vi "Host_ZConstantCurrentOscillation.vi"() -> ()   [LabVIEW 2014]
uses:
  <vilib>/Native 3D Graph/xcontrol/3DPC_SurfacePlot.xctl
  <vilib>/FPGAPlugInAG/PCIe-7851R/niLvFpga_Open_PCIe-7851R.vi
  <vilib>/rvi/interface/common/dynamic/niFpgaDynamicAddResources.vi
  <vilib>/Utility/error.llb/Error Cluster From Error Code.vi
  <vilib>/rvi/errors/niLvFpgaAdjustHostInterfaceError.vi
  <vilib>/FPGAPlugInAG/Dynamic/niLvFpga_Close_Dynamic.vi
  <vilib>/rvi/interface/nirviOpenFPGA/nirviOpenFPGA.xnode
  FPGA Bitfiles/PCCrossingZProje_FPGATarget_FPGAZAdjustment_qUJ-V0WWkAE.lvbitx
  <vilib>/rvi/interface/nirviReadWriteControl/nirviReadWriteControl.xnode
  <vilib>/rvi/interface/nirviMethod/nirviMethod.xnode
  <vilib>/rvi/interface/nirviCloseFPGA/nirviCloseFPGA.xnode
  NiFpgaLv.dll
  <vilib>/rvi/interface/Simulation/niFpgaSimulationCallBeginRW.vi
  <vilib>/FPGAPlugInAG/Dynamic/niLvFpga_ReadFifo_Dynamic.vi
  <vilib>/rvi/errors/niLvFpgaMergeErrorWithErrorCode.vi
panel:
  out "Connector0/DIO0":bool
  out "Connector0/DIO2":bool
  out "Connector0/DIO1":bool
  out "Elements Remaining":u32
  out "3D Graph":refnum<class "Base Datatype.lvclass">[](xcontrol)
  in  "YNum":i32
  in  "XNum":i32
  out "ZPos":i16(graph)
  in  "stop":bool
  in  "ZOffset index":i16
  # "Check with the XY part!"
  # "Check with the XY part!"
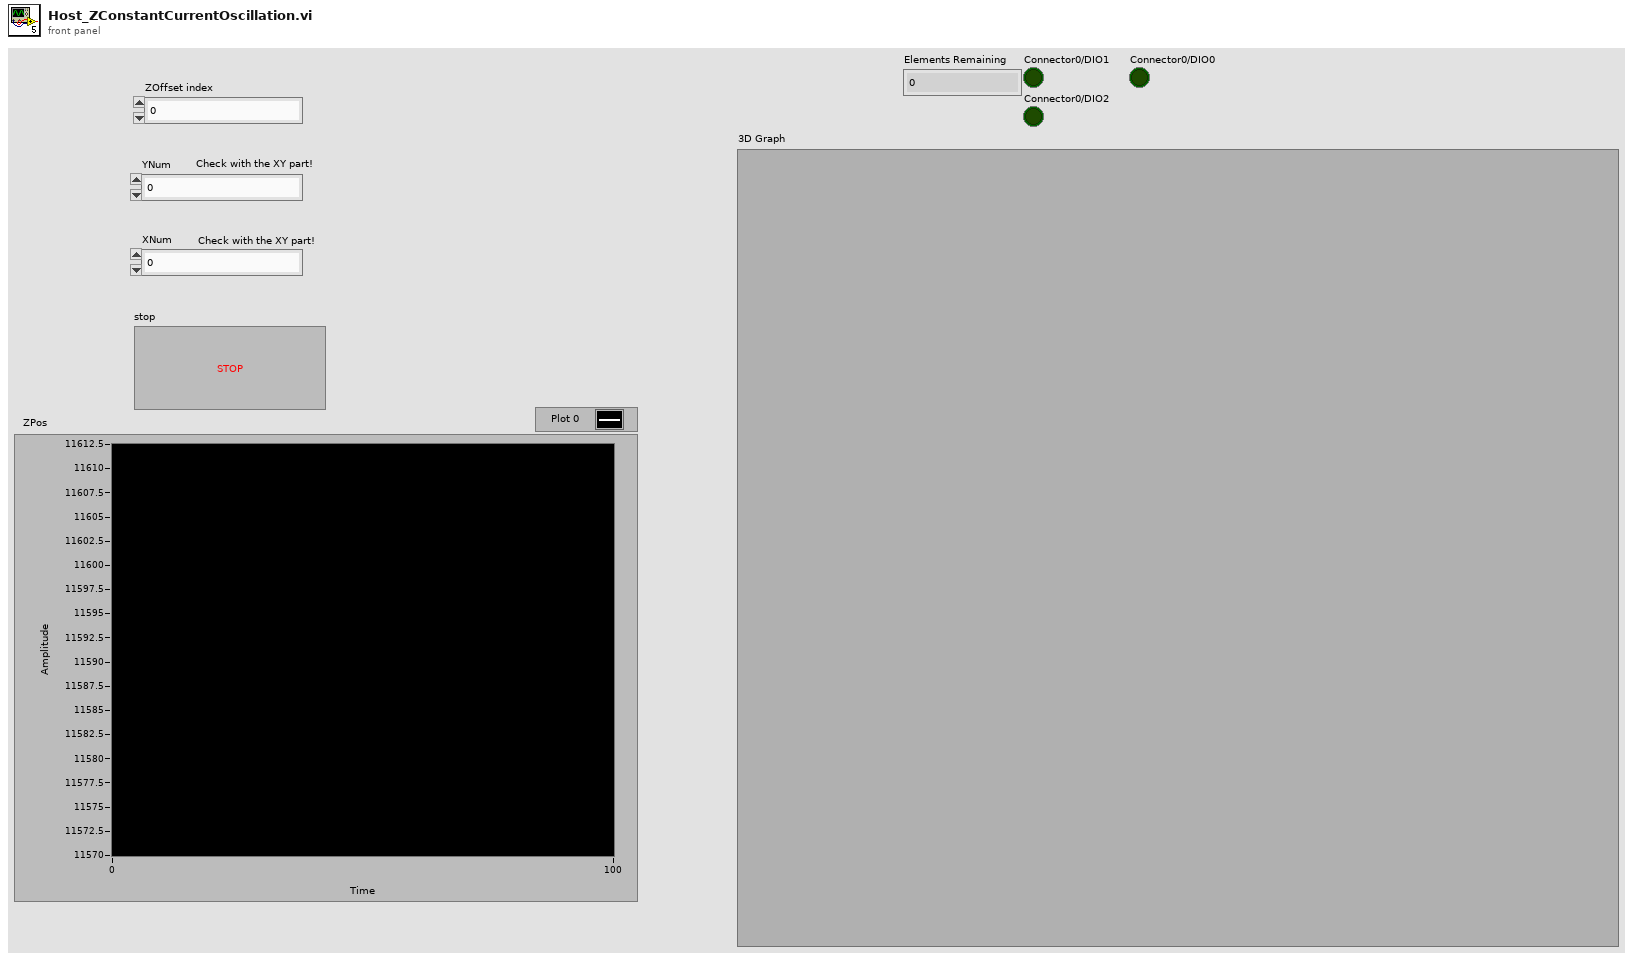
[diagram p1: front panel]
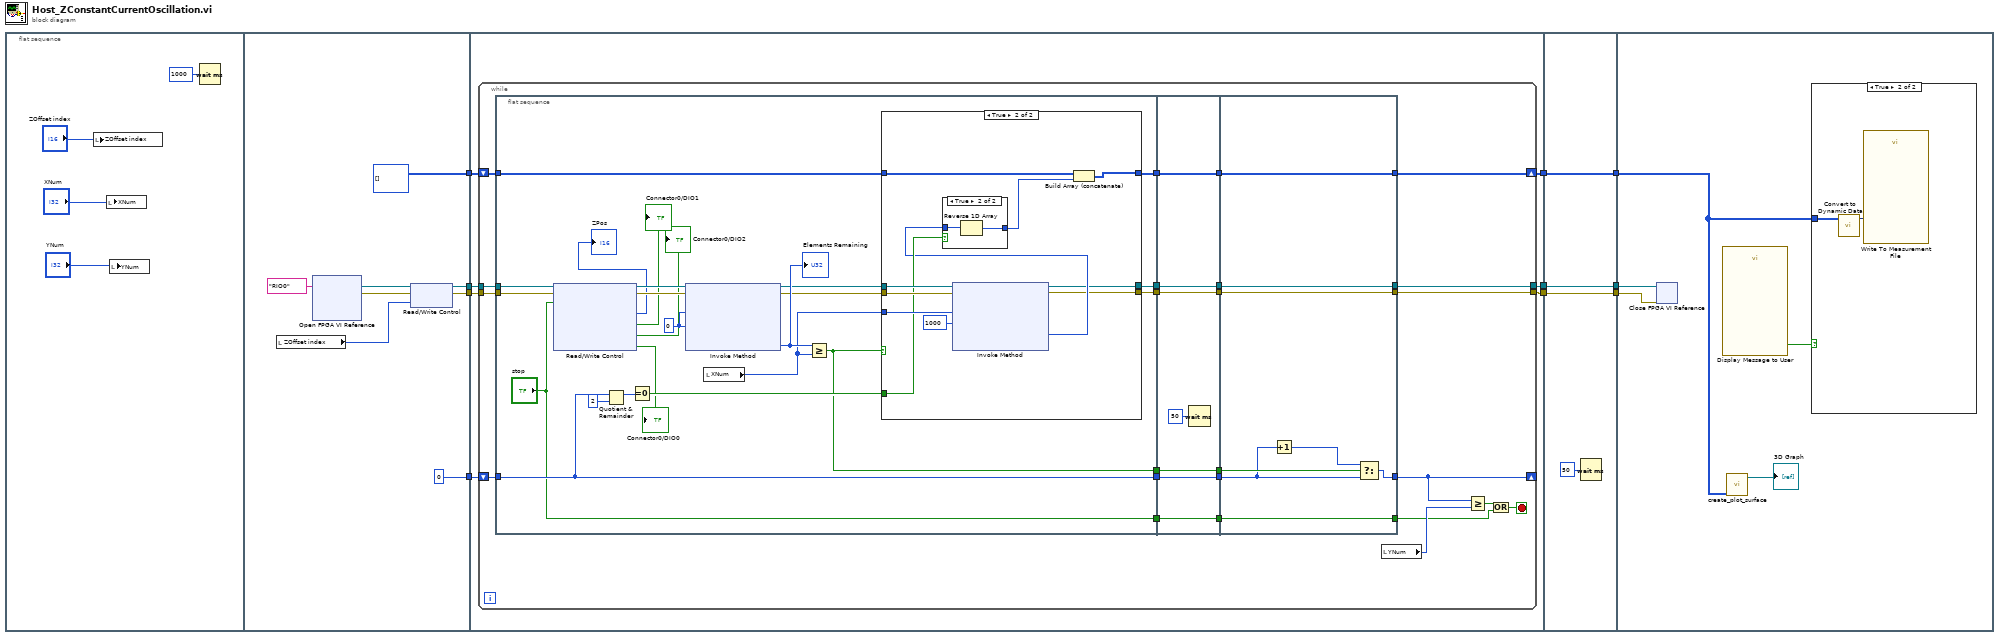
[diagram p0: block diagram]
diagram:
  n1 = flat-sequence {
    tunnel: [w19] -> w10
    tunnel: [w18] -> w9
    tunnel: [i16[][] []] -> w8
    tunnel: [0] -> w7
    tunnel: w10 -> [w28]
    tunnel: w9 -> [w27]
    tunnel: w8 -> [w29]
    tunnel: w7 -> [w26]
    tunnel: [w25] -> w6
    tunnel: [w24] -> w4
    tunnel: [w23] -> w2
    tunnel: w6 -> [w112]
    tunnel: [w112] -> w5
    tunnel: w4 -> [w111]
    tunnel: [w111] -> w3
    tunnel: w2 -> [w110]
    tunnel: [w110] -> w1
    tunnel: w5 -> [w115]
    tunnel: w3 -> [w116]
    tunnel: w1 -> [w113]
    frame #0 {
      n2 = local write "ZOffset index"("ZOffset index") -> ()
      n3 = local write "XNum"("XNum") -> ()
      n4 = local write "YNum"("YNum") -> ()
      n5 = Wait (ms)(milliseconds to wait=u32 1000) -> ()  [unwired: 1 out]
    }
    frame #1 {
      n6 = local read "ZOffset index"() -> (w15:i16)
      n7 = xnode ("Open FPGA VI Reference")("resource name"=tag "RIO0") -> ("FPGA VI Reference Out"=w21:refnum<k20>, "error out"=w20:errorcluster)  [unwired: 1 in]
      n8 = xnode "Read/Write Control"("FPGA VI Reference In"=w21, "error in"=w20, "ZOffset"=w15) -> ("FPGA VI Reference Out"=w19:refnum<k20>, "error out"=w18:errorcluster)
    }
    frame #2 {
      n9 = while {
        shift-right: [w49] -> w23
        shift-left: w29 -> [w53]
        tunnel: w28 -> [w52]
        tunnel: w27 -> [w51]
        shift-right: [w46] -> _
        shift-left: w26 -> [w50]
        tunnel: [w45] -> w25
        tunnel: [w44] -> w24
        stop <- w48 stop-if-true
        n10 = flat-sequence {
          tunnel: w53 -> [w63]
          tunnel: w52 -> [w76]
          tunnel: w51 -> [w75]
          tunnel: w50 -> [w59]
          tunnel: [w62] -> w41
          tunnel: [w61] -> w39
          tunnel: [w60] -> w37
          tunnel: [w59] -> w35
          tunnel: [w58] -> w33
          tunnel: ["stop"] -> w31
          tunnel: w41 -> [w100]
          tunnel: [w100] -> w40
          tunnel: w39 -> [w99]
          tunnel: [w99] -> w38
          tunnel: w37 -> [w98]
          tunnel: [w98] -> w36
          tunnel: w35 -> [w97]
          tunnel: [w97] -> w34
          tunnel: w33 -> [w96]
          tunnel: [w96] -> w32
          tunnel: w31 -> [w95]
          tunnel: [w95] -> w30
          tunnel: [w108] -> w49
          tunnel: w40 -> [w108]
          tunnel: w38 -> [w103]
          tunnel: w36 -> [w102]
          tunnel: w34 -> [w105]
          tunnel: w32 -> [w107]
          tunnel: [w104] -> w46
          tunnel: [w103] -> w45
          tunnel: [w102] -> w44
          tunnel: w30 -> [w101]
          tunnel: [w101] -> w42
          frame #0 {
            w71 = 0
            n11 = xnode "Read/Write Control"("FPGA VI Reference In"=w76, "error in"=w75, "stop"="stop") -> ("FPGA VI Reference Out"=w74:refnum<k20>, "error out"=w73:errorcluster, "ZRealTimePos"=→"ZPos":i16, "Connector0/DIO1"=→"Connector0/DIO1":bool, "Connector0/DIO2"=→"Connector0/DIO2":bool, "Connector0/DIO0"=→"Connector0/DIO0":bool)
            n12 = Quotient & Remainder(x=w59, y=2) -> (x-y*floor(x/y)=w68:i32)  [unwired: 1 out]
            n13 = Equal To 0?(x=w68) -> (x = 0?=w67:bool)
            n14 = xnode "Invoke Method"("FPGA VI Reference In"=w74, "error in"=w73, "Number of Elements"=w71, "Timeout (ms)"=w71) -> ("FPGA VI Reference Out"=w66:refnum<k20>, "error out"=w65:errorcluster, "Elements Remaining"=w70:u32)  [unwired: 1 out]
            "Elements Remaining" <- w70
            n15 = local read "XNum"() -> (w64:i32)
            n16 = Greater Or Equal?(x=w70, y=w64) -> (x >= y?=w58:bool)
            n17 = case shown="True" w58 {
              tunnel: w67 -> [_ w86]
              tunnel: w66 -> [w78 w90]
              tunnel: w65 -> [w77 w89]
              tunnel: w64 -> [_ w88]
              tunnel: w63 -> [w79 w84]
              tunnel: [w79 w82] -> w62
              tunnel: [w78 w81] -> w61
              tunnel: [w77 w80] -> w60
              frame False {
              }
              frame True {
                n18 = xnode "Invoke Method"("FPGA VI Reference In"=w90, "error in"=w89, "Number of Elements"=w88, "Timeout (ms)"=1000) -> ("FPGA VI Reference Out"=w81:refnum<k20>, "error out"=w80:errorcluster, "Data"=w85:i16[])  [unwired: 1 out]
                n19 = case shown="True" w86 {
                  tunnel: w85 -> [w91 w93]
                  tunnel: [w91 w92] -> w83
                  frame False {
                  }
                  frame True {
                    n20 = Reverse 1D Array(array=w93) -> (reversed array=w92:i16[])
                  }
                }
                n21 = Build Array (concatenate)(w84, w83) -> (w82:i16[][])
              }
            }
          }
          frame #1 {
            n22 = Wait (ms)(milliseconds to wait=u32 50) -> ()  [unwired: 1 out]
          }
          frame #2 {
            n23 = Increment(x=w105) -> (x+1=w106:i32)
            n24 = Select(t=w106, s=w107, f=w105) -> (s? t:f=w104:i32)
          }
        }
        n25 = local read "YNum"() -> (w43:i32)
        n26 = Greater Or Equal?(x=w46, y=w43) -> (x >= y?=w47:bool)
        n27 = Or(x=w47, y=w42) -> (x .or. y?=w48:bool)
      }
    }
    frame #3 {
      n28 = Wait (ms)(milliseconds to wait=u32 50) -> ()  [unwired: 1 out]
    }
    frame #4 {
      n29 = xnode "Close FPGA VI Reference"("FPGA VI Reference In"=w115, "error in"=w116) -> ()  [unwired: 1 out]
      n30 = call "Display Message to User"() -> ("OK"=w114:bool)  [unwired: 10 in, 1 out]
      n31 = call <vilib>:"create_plot_surface.vi"("z matrix"=w113) -> ("plots out"=→"3D Graph":refnum<class "Base Datatype.lvclass">[])  [unwired: 4 in, 6 out]
      n32 = case shown="True" w114 {
        tunnel: w113 -> [_ w119]
        frame False {
        }
        frame True {
          n33 = call "Convert to Dynamic Data"("2D Array"=w119) -> ("Dynamic Data Type"=w118:dynamicdata)  [unwired: 3 in]
          n34 = call "Write To Measurement File"("Signals"=w118) -> ()  [unwired: 16 in, 3 out]
        }
      }
    }
  }
